vi "Reset Alarms.vi"(0 "VISA resource name":refnum<visa-resource-name>, 7 "Reset Alarms (True)":bool=TRUE, 11 "error in (no error)":errorcluster) -> (4 "VISA resource name out":refnum<visa-resource-name>, 15 "error out":errorcluster)   [LabVIEW 2025, in "Lake Shore Cryotronics 370.lvlib"]
doc: "This VI clears both the high and low status of all alarms, including latching alarms."
uses:
  Lake Shore Cryotronics 370.lvlib
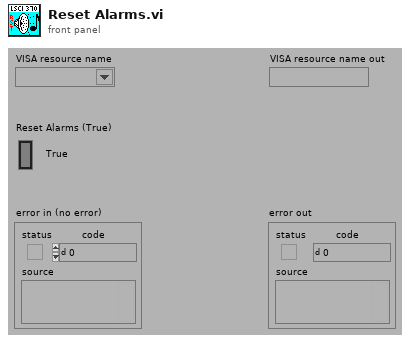
[diagram p1: front panel]
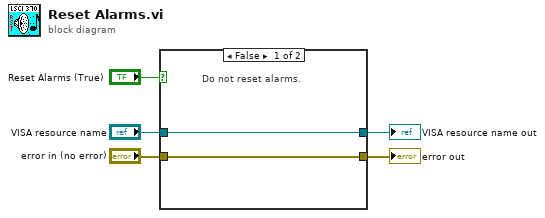
[diagram p0: block diagram]
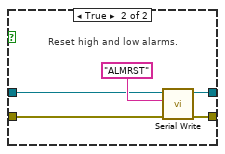
[diagram p2: hidden frame]
diagram:
  n1 = case shown="False" "Reset Alarms (True)" {
    tunnel: "VISA resource name" -> [w7 w11]
    tunnel: "error in (no error)" -> [w6 w10]
    tunnel: [w6 w9] -> w2
    tunnel: [w7 w8] -> w1
    frame False {
      # "Do not reset alarms."
    }
    frame True {
      # "Reset high and low alarms."
      n2 = call "Serial Write.vi"("error in (no error)"=w10, "Write Buffer (\"\")"="ALMRST", "VISA resource name"=w11) -> ("error out"=w9:errorcluster, "VISA resource name out"=w8:refnum<visa-resource-name>)  [unwired: 6 in, 1 out]
    }
  }
  "error out" <- w2
  "VISA resource name out" <- w1
